vi "Concat Data.vi"(0 "AKLH Today Dirs":path[](array[path]), 1 "Concat Data":bool, 5 "AKLH Sync Dirs":path[](array[path]), 7 "AKLH Dirs":path[](array[path]), 9 "AKLH Today Hdr Paths":path[](array[path]), 11 "AKLH Filenames":string[](array[string])) -> ()   [LabVIEW 2013]
uses:
  <vilib>/Utility/file.llb/Read From Spreadsheet File (DBL).vi
  <vilib>/Utility/file.llb/Write To Spreadsheet File (DBL).vi
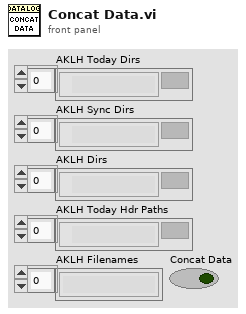
[diagram p1: front panel]
types:
  T1 = typedef "LVDateTimeRec.ctl" = cluster{"fractional second":dbl, "second":i32, "minute":i32, "hour":i32, "day of month":i32, "month":i32, "year":i32, "day of week":i32, "day of year":i32, "DST":i32}
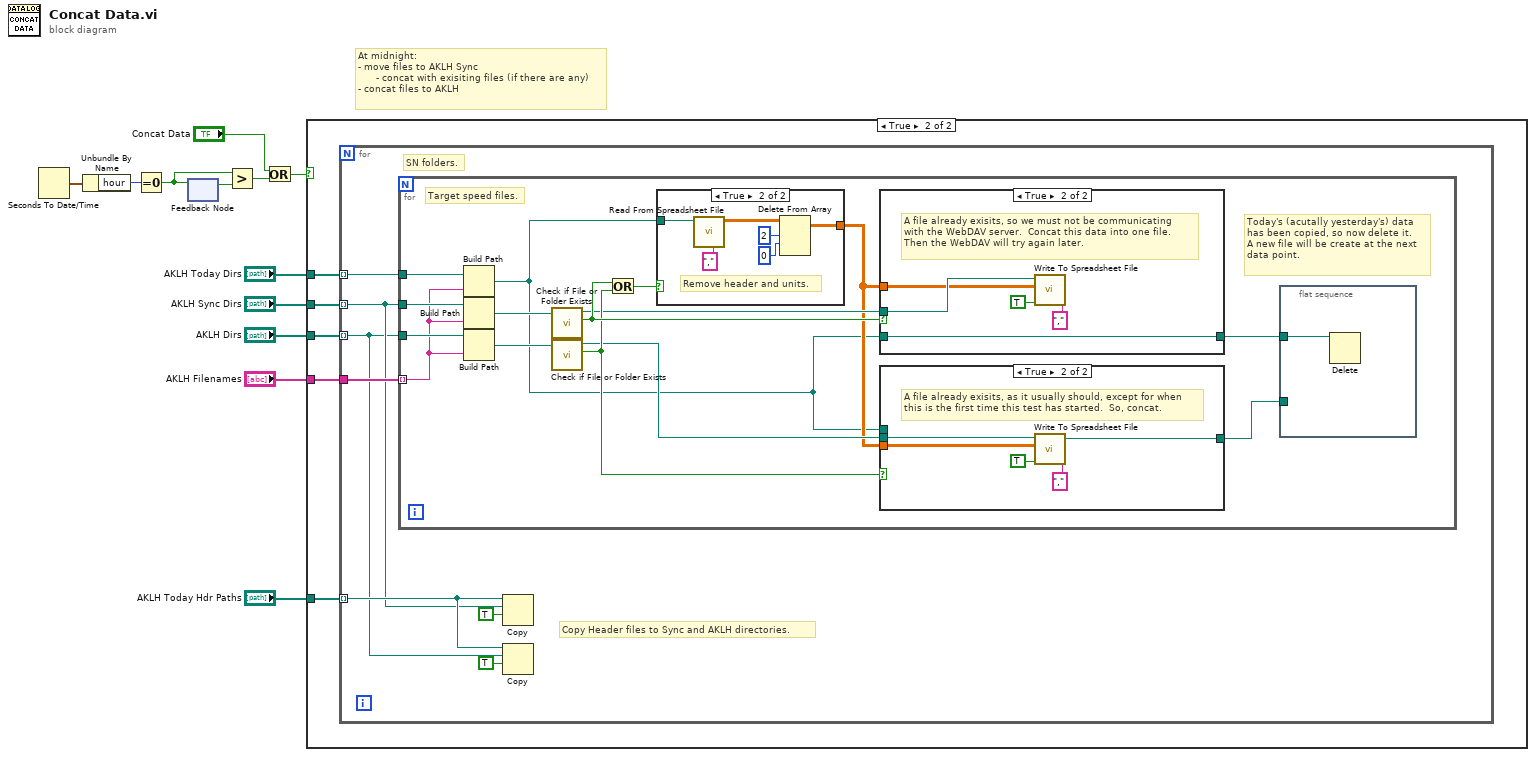
[diagram p0: block diagram]
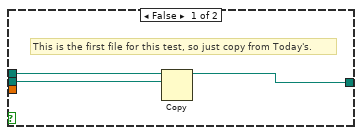
[diagram p3: hidden frame]
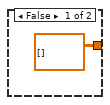
[diagram p4: hidden frame]
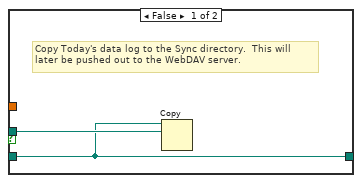
[diagram p5: hidden frame]
diagram:
  # "At midnight:\n- move files to AKLH Sync\n      - concat with exisiting files (if there are any)\n- concat files to AKLH"
  n1 = Seconds To Date/Time() -> (date time rec=w12:T1)  [unwired: 2 in]
  n2 = Unbundle By Name(w12) -> ("hour"=w2:i32)
  n3 = Equal To 0?(x=w2) -> (x = 0?=w1:bool)
  n4 = feedback-in #1(w1) -> ()
  n5 = feedback #1() -> (w11:bool)  [unwired: 1 in]
  n6 = Greater?(x=w1, y=w11) -> (0:w5:bool)
  n7 = Or(x="Concat Data", y=w5) -> (x .or. y?=w4:bool)
  n8 = case shown="True" w4 {
    tunnel: "AKLH Today Dirs" -> [_ w17]
    tunnel: "AKLH Sync Dirs" -> [_ w16]
    tunnel: "AKLH Dirs" -> [_ w15]
    tunnel: "AKLH Filenames" -> [_ w14]
    tunnel: "AKLH Today Hdr Paths" -> [_ w13]
    frame False {
    }
    frame True {
      n9 = for {
        tunnel: w17 -> [w24] mode=indexing
        tunnel: w16 -> [w19] mode=indexing
        tunnel: w15 -> [w18] mode=indexing
        tunnel: w14 -> [w23]
        tunnel: w13 -> [w20] mode=indexing
        # "Copy Header files to Sync and AKLH directories."
        # "SN folders."
        n10 = for {
          tunnel: w24 -> [w39]
          tunnel: w19 -> [w38]
          tunnel: w18 -> [w37]
          tunnel: w23 -> [w36] mode=indexing
          # "Today's (acutally yesterday's) data\nhas been copied, so now delete it.\nA new file will be create at the next\ndata point."
          # "Target speed files."
          n11 = Build Path(base path=w39, name or relative path=w36) -> (appended path=w27:path)
          n12 = Build Path(base path=w38, name or relative path=w36) -> (appended path=w35:path)
          n13 = Build Path(base path=w37, name or relative path=w36) -> (appended path=w34:path)
          n14 = call <vilib>:"Check if File or Folder Exists.vi"("path"=w35) -> ("file or folder exists?"=w32:bool, "dup path"=w30:path)  [unwired: 8 in, 1 out]
          n15 = call <vilib>:"Check if File or Folder Exists.vi"("path"=w34) -> ("file or folder exists?"=w31:bool, "dup path"=w29:path)  [unwired: 8 in, 1 out]
          n16 = Or(x=w32, y=w31) -> (x .or. y?=w33:bool)
          n17 = case shown="True" w33 {
            tunnel: w27 -> [_ w51]
            tunnel: [dbl[][] [] ("all rows") w50] -> w28
            frame False {
            }
            frame True {
              # "Remove header and units."
              n18 = call-poly <vilib>:"Read From Spreadsheet File.vi"("delimiter (\\t)"="," ("delimiter (\\t)"), "file path (dialog if empty)"=w51) -> ("all rows"=w54:dbl[][])  [unwired: 5 in, 4 out]
              n19 = Delete From Array(array=w54, length=2, index (row)=0) -> (array with subset deleted=w50:dbl[][])  [unwired: 1 in, 1 out]
            }
          }
          n20 = case shown="True" w32 {
            tunnel: w30 -> [w57 w60]
            tunnel: w28 -> [_ w59]
            tunnel: w27 -> [w56 w58]
            tunnel: [w56 w58] -> w25
            frame False {
              # "Copy Today's data log to the Sync directory.  This will\nlater be pushed out to the WebDAV server."
              n21 = Copy(10:w57, 11:w56) -> ()  [unwired: 3 in, 3 out]
            }
            frame True {
              # "A file already exisits, so we must not be communicating\nwith the WebDAV server.  Concat this data into one file.\nThen the WebDAV will try again later."
              n22 = call-poly <vilib>:"Write To Spreadsheet File.vi"("delimiter (\\t)"="," ("delimiter (\\t)"), "append to file? (new file:F)"=TRUE, "2D data"=w59, "file path (dialog if empty)"=w60) -> ()  [unwired: 4 in, 1 out]
            }
          }
          n23 = case shown="True" w31 {
            tunnel: w29 -> [w42 w46]
            tunnel: w28 -> [_ w45]
            tunnel: w27 -> [w43 _]
            tunnel: [w41 w44] -> w26
            frame False {
              # "This is the first file for this test, so just copy from Today's."
              n24 = Copy(10:w42, 11:w43) -> (3:w41:path)  [unwired: 3 in, 2 out]
            }
            frame True {
              # "A file already exisits, as it usually should, except for when\nthis is the first time this test has started.  So, concat."
              n25 = call-poly <vilib>:"Write To Spreadsheet File.vi"("delimiter (\\t)"="," ("delimiter (\\t)"), "append to file? (new file:F)"=TRUE, "2D data"=w45, "file path (dialog if empty)"=w46) -> ("new file path (Not A Path if cancelled)"=w44:path)  [unwired: 4 in]
            }
          }
          n26 = flat-sequence {
            tunnel: w26 -> [_]
            tunnel: w25 -> [w40]
            frame #0 {
              n27 = Delete(path (use dialog)=w40) -> ()  [unwired: 4 in, 3 out]
            }
          }
        }
        n28 = Copy(9:TRUE ("overwrite (F)"), 10:w19, 11:w20) -> ()  [unwired: 2 in, 3 out]
        n29 = Copy(9:TRUE ("overwrite (F)"), 10:w18, 11:w20) -> ()  [unwired: 2 in, 3 out]
      }
    }
  }
